vi "TestDataLink.vi"() -> (0 "Error":bool)   [LabVIEW 2014]
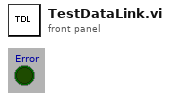
[diagram p1: front panel]
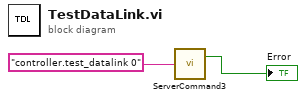
[diagram p0: block diagram]
diagram:
  n1 = call "ServerCommand3.vi"("Command"="controller.test_datalink 0") -> ("Error"=→"Error":bool)  [unwired: 1 out]
